vi "Run Slam (SubVI).vi"(6 "slam itearations":i32=4, 9 "Lidar Offset from Center of Rotation (mm)":dbl=100.0 format="%#_13g", 10 "Lidar Data":T1, 11 "Library Path":path) -> (3 "Pose Delta":cluster{"X":dbl, "Y":dbl, "R":dbl})   [LabVIEW 2017]
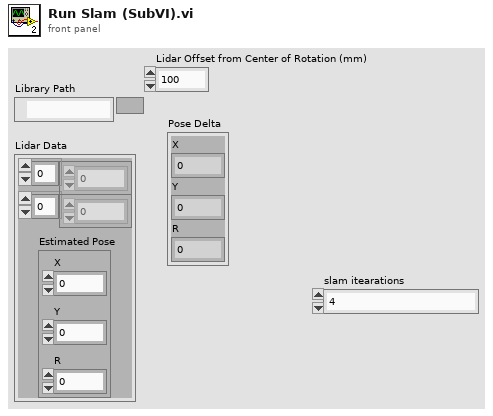
[diagram p1: front panel]
types:
  T1 = cluster{dbl[], dbl[], "Estimated Pose":cluster{"X":dbl, "Y":dbl, "R":dbl}}
  T2 = cluster{"ets_x":dbl, "est_y":dbl, "est_theta":dbl}
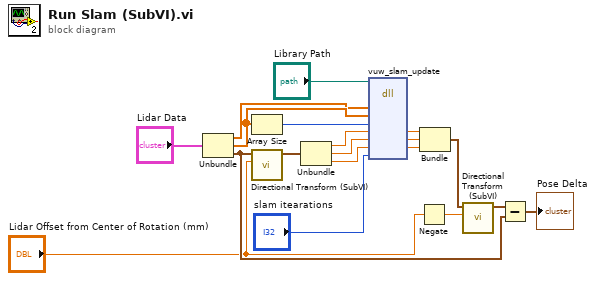
[diagram p0: block diagram]
diagram:
  n1 = Unbundle("Lidar Data") -> (w11:dbl[], w12:dbl[], "Estimated Pose"=w3:cluster{"X":dbl, "Y":dbl, "R":dbl})
  n2 = Array Size(array=w12) -> (size(s)=w8:i32)
  n3 = call "Directional Transform (SubVI).vi"("Transform Amount (mm)"="Lidar Offset from Center of Rotation (mm)", "Pose"=w3) -> ("Pose"=w4:cluster{"X":dbl, "Y":dbl, "R":dbl})  [unwired: 9 in]
  n4 = Unbundle(w4) -> ("X"=w14:dbl, "Y"=w15:dbl, "R"=w18:dbl)
  n5 = dll-call lib="?" fn="vuw_slam_update"(path in="Library Path", "x"=w11, "y"=w12, "nb_points"=w8, "ets_x"=w14, "est_y"=w15, "est_theta"=w18, "itearations"="slam itearations") -> ("ets_x"=w16:dbl, "est_y"=w17:dbl, "est_theta"=w19:dbl)  [unwired: 7 in, 2 out]
  n6 = Negate(x="Lidar Offset from Center of Rotation (mm)") -> (-x=w2:dbl)
  n7 = Bundle("ets_x"=w16, "est_y"=w17, "est_theta"=w19) -> (w6:T2)  [unwired: 1 in]
  n8 = call "Directional Transform (SubVI).vi"("Transform Amount (mm)"=w2, "Pose"=w6) -> ("Pose"=w5:cluster{"X":dbl, "Y":dbl, "R":dbl})  [unwired: 9 in]
  n9 = Subtract(x=w5, y=w3) -> (x-y=→"Pose Delta":cluster{"X":dbl, "Y":dbl, "R":dbl})
